vi "Receive String Value Msg.vi"(8 "error in (no error)":errorcluster, 10 "StringValueMsg":refnum<class "StringValueMsg.lvclass">, 11 "IController In":refnum<class "IController.lvclass">) -> (0 "error out":errorcluster, 3 "IController Out":refnum<class "IController.lvclass">)   [LabVIEW 2015, in "IController.lvlib" / "IController.lvclass"]
uses:
  IController.lvclass
  AutoRegistration/ActorAutoRegistration Messages/StringValueMsg/StringValueMsg.lvclass
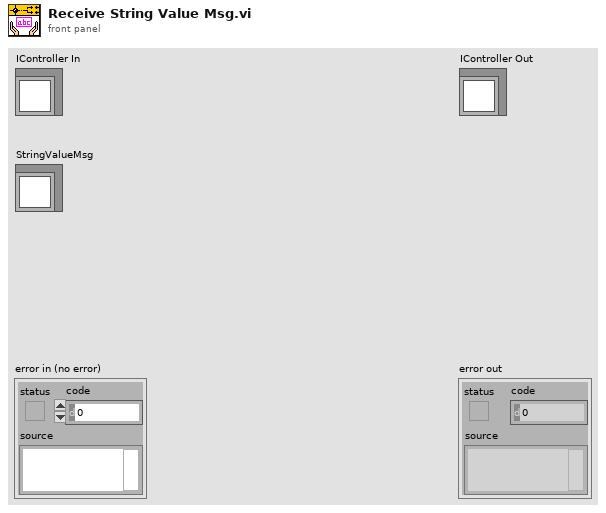
[diagram p1: front panel]
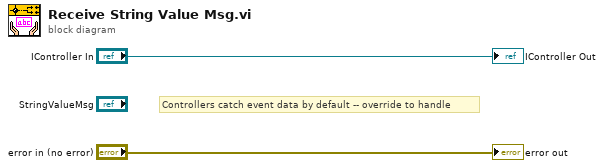
[diagram p0: block diagram]
diagram:
  # "Controllers catch event data by default -- override to handle"
  "error out" <- "error in (no error)"
  "IController Out" <- "IController In"
